vi "dsc9513ReadHoldRegister.vi"(8 "error in":errorcluster, 10 "counter":u8=1 min=1 max=10, 11 "board":i16) -> (0 "error out":errorcluster, 1 "value":u16, 2 "counter_out":u8, 3 "boardOut":i16)   [LabVIEW 2011, in "Diamond Universal Driver.lvlib"]
doc: "This function returns the 16-bit data in the selected counter's hold register. The counter data must first be latched by a Save or Save and Disarm command using dsc9513CounterControl() or dsc9513SingleCounterControl()."
uses:
  Diamond Universal Driver.lvlib
  Controls/error codes.ctl
  Instruments/WL OPC/Support/dlls/dscud.dll
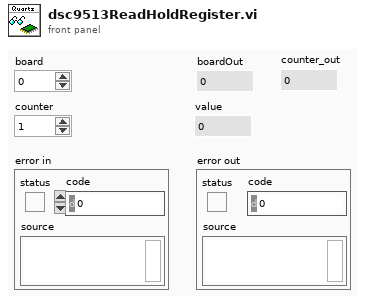
[diagram p1: front panel]
types:
  T1 = typedef "Diamond Universal Driver.lvlib/error codes.ctl" = enum8{"DE_NONE", "DE_HW_FAILURE", "DE_SW_FAILURE", "DE_HW_NOT_SUPPORTED", "DE_SW_NOT_SUPPORTED", "DE_INVALID_PARM", "DE_ALTERNATE_IN_PROGRESS", "DE_NONE_IN_PROGRESS", "DE_BUFFER_ROLLOVER", "DE_INVALID_ERROR_CODE", "DE_ALREADY_PAUSED", "DE_OVERFLOW", "DE_INVALID_FUNC", "DE_DSCUDH_INVALID", "DE_INVALID_BOARD", "DE_BOARD_LIMIT_REACHED", "DE_BOARD_BUSY", "DE_INVALID_WINDRVR_HANDLE", "DE_INVALID_WINDRVR_VERSION", "DE_BAD_WINDRVR_BOARD_INIT", "DE_OPERATION_TIMED_OUT", "DE_INVALID_WINDRVR_KP", "DE_THREAD_FAILURE"}
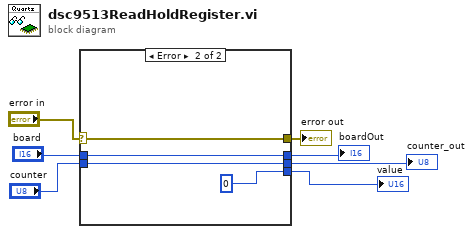
[diagram p0: block diagram]
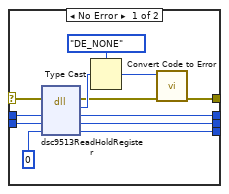
[diagram p2: hidden frame]
diagram:
  n1 = case shown="Error" "error in" {
    selector: "error in" -> [w16 w23]
    tunnel: "board" -> [w14 w22]
    tunnel: [w13 w22] -> w5
    tunnel: [w12 w23] -> w4
    tunnel: "counter" -> [w11 w20]
    tunnel: [w9 u16 0 ("value")] -> w2
    tunnel: [w8 w20] -> w1
    frame No Error {
      n2 = dll-call lib="C:/Users/mrichardson/Documents/Web Based Version Control SW/Instruments/WL OPC/Support/dlls/dscud.dll" fn="dsc9513ReadHoldRegister"(error in=w16, "board"=w14, "counter"=w11, "value"=u16 0) -> (error out=w15:errorcluster, "error"=w17:u8, "board"=w13:i16, "counter"=w8:u8, "value"=w9:u16)  [unwired: 2 in, 1 out]
      n3 = Type Cast(type=error_codes."DE_NONE" ("error codes"), x=w17) -> (*(type *) &x=w19:T1)
      n4 = call "Convert Code to Error.vi"("error in"=w15, "error codes"=w19) -> ("error out"=w12:errorcluster)  [unwired: 9 in]
    }
    frame Error {
    }
  }
  "boardOut" <- w5
  "error out" <- w4
  "value" <- w2
  "counter_out" <- w1
